vi "GetBigDigit.vi"(8 "error in (no error)":errorcluster, 10 "Digit":i32, 11 "color":fxp<+,3,3>) -> (0 "error out":errorcluster, 3 "Array":u32[][](array[numeric]))   [LabVIEW 2019, in "RT_Game.lvlib" / "Game.lvclass"]
uses:
  Game.lvclass
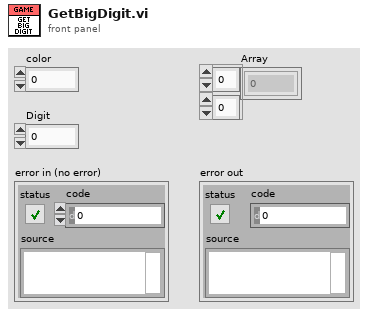
[diagram p1: front panel]
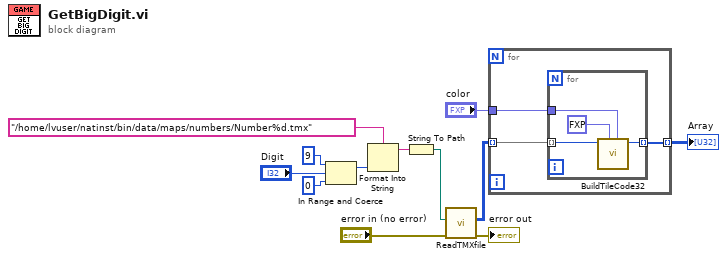
[diagram p0: block diagram]
diagram:
  n1 = In Range and Coerce(upper limit=9, x="Digit", lower limit=0) -> (coerced(x)=w3:i32)  [unwired: 1 out]
  n2 = Format Into String(format string="/home/lvuser/natinst/bin/data/maps/numbers/Number%d.tmx" ("path to tmx-file (created with Tiles2D)"), w3) -> (resulting string=w8:string)  [unwired: 2 in, 1 out]
  n3 = String To Path(string=w8) -> (path=w11:path)
  n4 = call "ReadTMXfile.vi"("error in (no error)"="error in (no error)", "path to tmx-file (created with Tiles2D)"=w11) -> ("error out"=→"error out":errorcluster, "Tilenumbers"=w10:u32[][])  [unwired: 8 in]
  n5 = for {
    tunnel: w10 -> [w15] mode=indexing
    tunnel: [w14] -> w12 mode=indexing
    tunnel: "color" -> [w13]
    n6 = for {
      tunnel: w15 -> [w19] mode=indexing
      tunnel: [w18] -> w14 mode=indexing
      tunnel: w13 -> [w16]
      n7 = call "BuildTileCode32.vi"("replacecolor"=w16, "color_to_replace"=fxp<+,3,3> 7.0, "Tilenumber"=w19) -> ("TileCode"=w18:u32)  [unwired: 8 in]
    }
  }
  "Array" <- w12
